vi "Ref Est.vi"(10 "IA State Input":T2) -> (1 "IA command":T1, 2 "IA State Output":T2)   [LabVIEW 2017]
uses:
  Command Enum.ctl
  Core/AI Ball.ctl
  Core/AI Judge.ctl
  Functions Enum.ctl
  Core/AI Robot.ctl
  Core/Field Size.ctl
  Core/AI Input.ctl
  AttackerStates.ctl
  Util/Events/Events.ctl
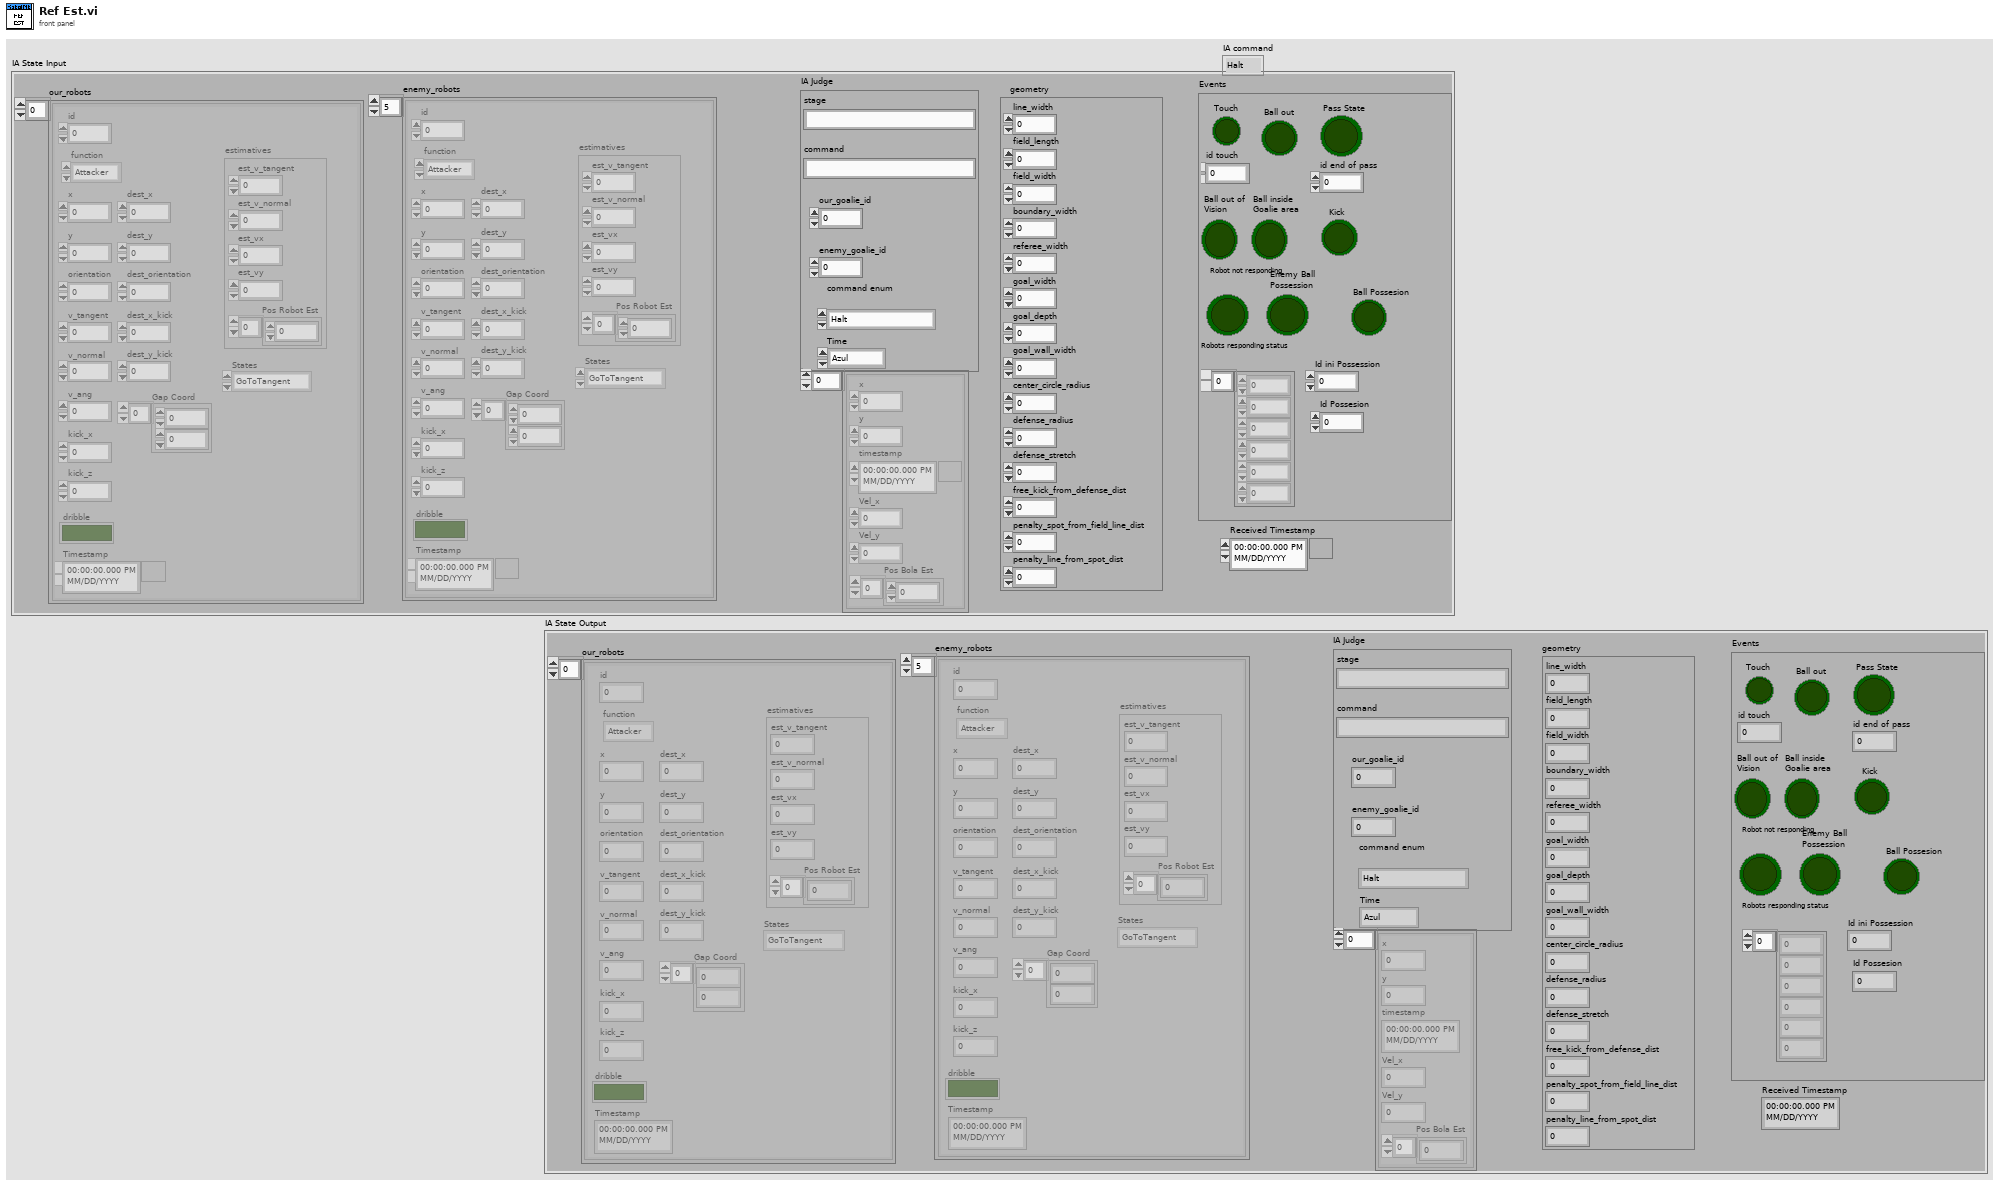
[diagram p1: front panel]
types:
  T1 = typedef "Command Enum.ctl" = enum16{"Halt", "Stop", "Force Start", "PKA Normal Start", "Prepare Kickoff Ally", "PKE Normal Start", "Prepare Kickoff Enemy", "Prepare Penalty Ally", "PPA Normal Start", "Prepare Penalty Enemy", "PPE Normal Start", "Direct Free Enemy", "Direct Free Ally", "Indirect Free Enemy", "Indirect Free Ally", "Timeout Enemy", "Timeout Ally", "Goal Enemy", "Goal Ally", "Ball Placement Enemy", "Ball Placement Ally", "Normal Half Time", "Extra Time Break", "Extra Half Time", "None", "Post Game"}
  T2 = typedef "AI Input.ctl" = cluster{"our_robots":T3[], "enemy_robots":T3[], "balls":T6[], "geometry":T7, "IA Judge":T8, "Received Timestamp":timestamp, "Events":T9}
  T3 = typedef "AI Robot.ctl" = cluster{"id":u32, "function":T4, "x":dbl, "y":dbl, "orientation":dbl, "v_tangent":dbl, "v_normal":dbl, "v_ang":dbl, "kick_x":dbl, "kick_z":dbl, "dribble":bool, "Timestamp":timestamp, "dest_x":dbl, "dest_y":dbl, "dest_orientation":dbl, "estimatives":cluster{"est_v_tangent":dbl, "est_v_normal":dbl, "est_vx":dbl, "est_vy":dbl, "Pos Robot Est":dbl[]}, "dest_x_kick":dbl, "dest_y_kick":dbl, "Gap Coord":dbl[], "States":T5}
  T4 = typedef "Functions Enum.ctl" = enum16{"Attacker", "Goalie", "Defender", "Striker", "Goto 0", "Dummy", "Kicker", "ZigZag"}
  T5 = typedef "AttackerStates.ctl" = enum16{"Pass", "GoToTangent", "BallGetting", "GoToKick", ""}
  T6 = typedef "AI Ball.ctl" = cluster{"x":dbl, "y":dbl, "timestamp":timestamp, "Vel_x":dbl, "Vel_y":dbl, "Pos Bola Est":dbl[]}
  T7 = typedef "Field Size.ctl" = cluster{"line_width":u32, "field_length":u32, "field_width":u32, "boundary_width":u32, "referee_width":u32, "goal_width":u32, "goal_depth":u32, "goal_wall_width":u32, "center_circle_radius":u32, "defense_radius":u32, "defense_stretch":u32, "free_kick_from_defense_dist":u32, "penalty_spot_from_field_line_dist":u32, "penalty_line_from_spot_dist":u32}
  T8 = typedef "AI Judge.ctl" = cluster{"stage":string, "command":string, "our_goalie_id":dbl, "enemy_goalie_id":dbl, "command enum":T1, "Time":enum16{"Azul", "Amarelo"}}
  T9 = typedef "Events.ctl" = cluster{"Touch":bool, "Ball out":bool, "id touch":dbl, "Ball out of \nVision":bool, "Ball inside \nGoalie area":bool, "Robot not responding":bool, "Robots responding status":dbl[], "Enemy Ball \nPossession":bool, "Pass State":bool, "id end of pass":dbl, "Kick":bool, "Id ini Possession":dbl, "Ball Possesion":bool, "Id Possesion":dbl}
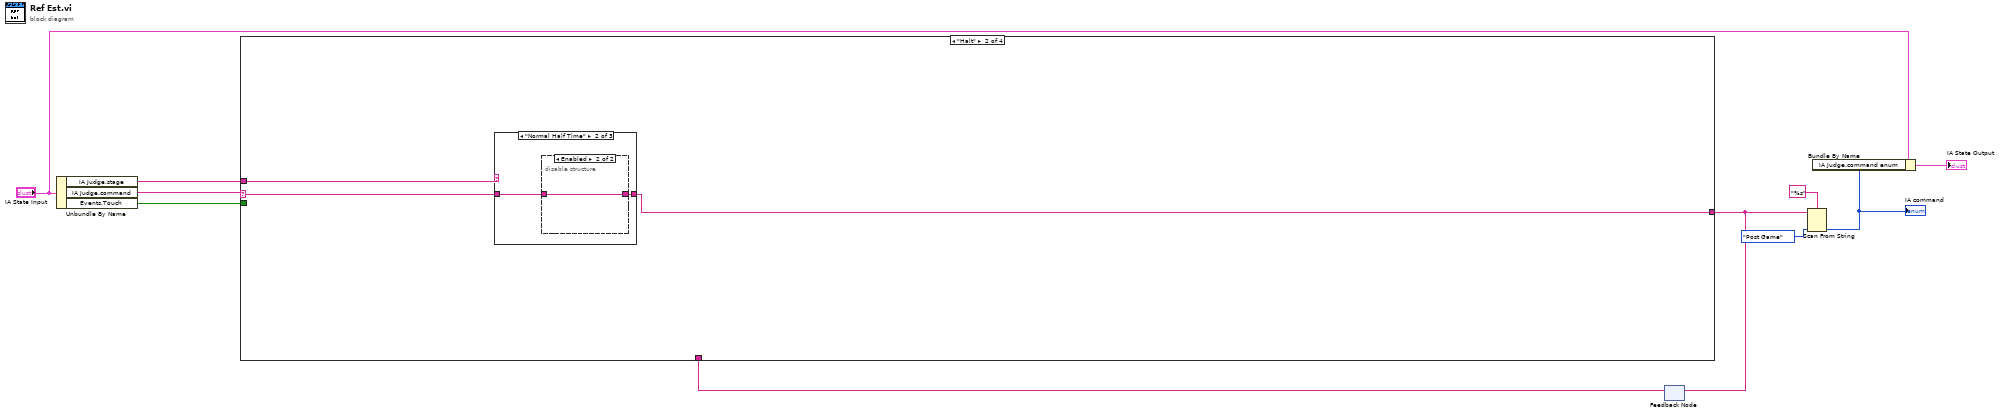
[diagram p0: block diagram]
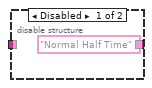
[diagram p4: hidden frame]
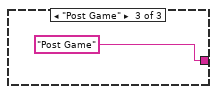
[diagram p5: hidden frame]
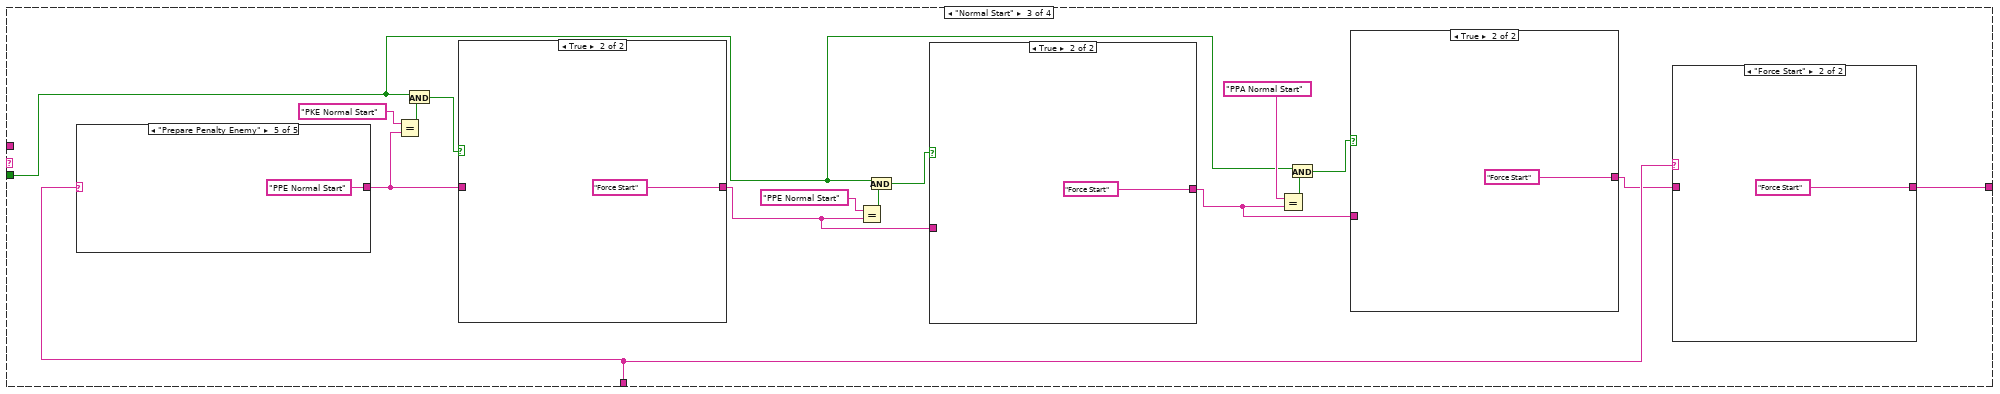
[diagram p6: hidden frame]
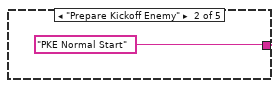
[diagram p12: hidden frame]
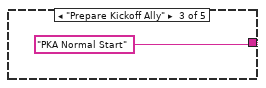
[diagram p13: hidden frame]
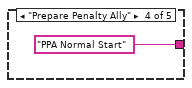
[diagram p14: hidden frame]
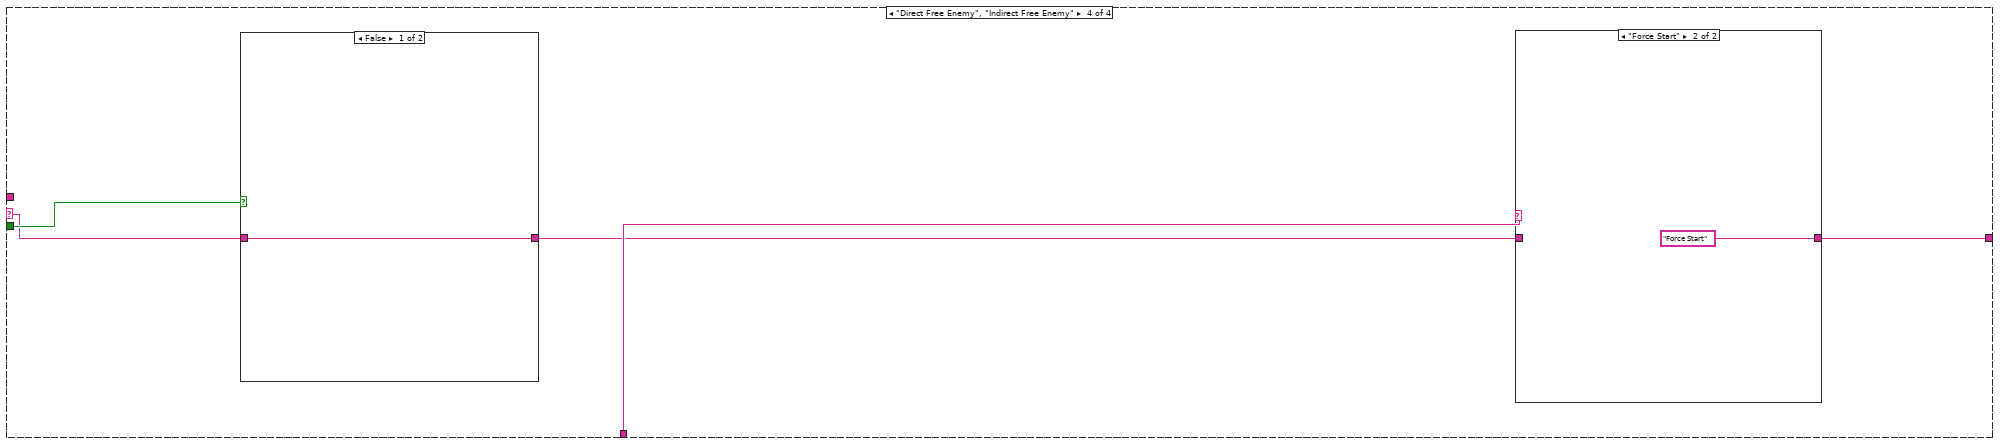
[diagram p15: hidden frame]
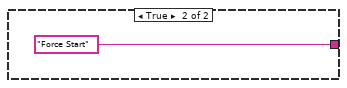
[diagram p17: hidden frame]
diagram:
  n1 = Unbundle By Name("IA State Input") -> ("IA Judge.stage"=w2:string, "IA Judge.command"=w10:string, "Events.Touch"=w4:bool)
  n2 = feedback #1() -> (w5:string)  [unwired: 1 in]
  n3 = case shown="\"Halt\"" w10 {
    selector: w10 -> [w11 w13 _ w53]
    tunnel: [w11 w12 w36 w51] -> w3
    tunnel: w5 -> [_ _ w35 w52]
    tunnel: w4 -> [_ _ w21 w54]
    tunnel: w2 -> [_ w14 _ _]
    frame Default {
    }
    frame "Halt" {
      n4 = case shown="\"Normal Half Time\"" w14 {
        tunnel: [w15 w17 "Post Game"] -> w12
        tunnel: w13 -> [w15 w16 _]
        frame Default {
        }
        frame "Normal Half Time" {
          n5 = disable-structure shown="Enabled" {
            disable-tunnel: ["Normal Half Time" w19] -> w17
            disable-tunnel: w16 -> [_ w19]
            frame Disabled {
            }
            frame Enabled {
            }
          }
        }
        frame "Post Game" {
        }
      }
    }
    frame "Normal Start" {
      n6 = case shown="\"Prepare Penalty Enemy\"" w35 {
        selector: w35 -> [w45 _ _ _ _]
        tunnel: [w45 "PKE Normal Start" "PKA Normal Start" "PPA Normal Start" "PPE Normal Start"] -> w33
        frame Default {
        }
        frame "Prepare Kickoff Enemy" {
        }
        frame "Prepare Kickoff Ally" {
        }
        frame "Prepare Penalty Ally" {
        }
        frame "Prepare Penalty Enemy" {
        }
      }
      n7 = Equal?(x="PKE Normal Start", y=w33) -> (x = y?=w34:bool)
      n8 = And(x=w21, y=w34) -> (x .and. y?=w23:bool)
      n9 = case shown="True" w23 {
        tunnel: [w43 "Force Start"] -> w28
        tunnel: w33 -> [w43 _]
        frame False {
        }
        frame True {
        }
      }
      n10 = Equal?(x="PPE Normal Start", y=w28) -> (x = y?=w31:bool)
      n11 = And(x=w21, y=w31) -> (x .and. y?=w29:bool)
      n12 = case shown="True" w29 {
        tunnel: [w39 "Force Start"] -> w24
        tunnel: w28 -> [w39 _]
        frame False {
        }
        frame True {
        }
      }
      n13 = Equal?(x="PPA Normal Start", y=w24) -> (x = y?=w27:bool)
      n14 = And(x=w21, y=w27) -> (x .and. y?=w25:bool)
      n15 = case shown="True" w25 {
        tunnel: [w37 "Force Start"] -> w22
        tunnel: w24 -> [w37 _]
        frame False {
        }
        frame True {
        }
      }
      n16 = case shown="\"Force Start\"" w35 {
        tunnel: [w41 "Force Start"] -> w36
        tunnel: w22 -> [w41 _]
        frame Default {
        }
        frame "Force Start" {
        }
      }
    }
    frame "Direct Free Enemy", "Indirect Free Enemy" {
      n17 = case shown="False" w54 {
        tunnel: [w57 "Force Start"] -> w50
        tunnel: w53 -> [w57 _]
        frame False {
        }
        frame True {
        }
      }
      n18 = case shown="\"Force Start\"" w52 {
        tunnel: [w55 "Force Start"] -> w51
        tunnel: w50 -> [w55 _]
        frame Default {
        }
        frame "Force Start" {
        }
      }
    }
  }
  n19 = feedback-in #1(w3) -> ()
  n20 = Scan From String(format string="%s", input string=w3, default 1=Command_Enum."Post Game" ("command\nenum")) -> (output 1=w7:T1)  [unwired: 2 in, 3 out]
  "IA command" <- w7
  n21 = Bundle By Name(cluster="IA State Input", "IA Judge.command enum"=w7) -> (→"IA State Output":T2)
